vi "Test Sampling.vi"(8 "error in (no error)":errorcluster, 11 "Instrument.Lockin in":refnum<class "Instrument.Lockin.lvclass">) -> (0 "error out":errorcluster, 3 "Instrument.Lockin out":refnum<class "Instrument.Lockin.lvclass">)   [LabVIEW 2016]
uses:
  src/Instrument.Lockin/Instrument.Lockin.lvclass
  src/LockinDAQ/Typedefs/Sampling.ctl
  <vilib>/addons/_JKI Toolkits/Caraya/classes/Assert/Assert Equal Value_Variant.vi
  <userlib>/_OpenG.lib/numeric/numeric.llb/Random Number Within Range - DBL__ogtk.vi
  <vilib>/addons/_JKI Toolkits/Caraya/classes/Assert/Assert Equal Value and Type_Variant.vi
  <vilib>/addons/_JKI Toolkits/Caraya/classes/Test/Test.lvclass
  src/LockinDAQ/LockinDAQ.lvclass
  <vilib>/addons/_JKI Toolkits/Caraya/classes/Assert/Assert.lvclass
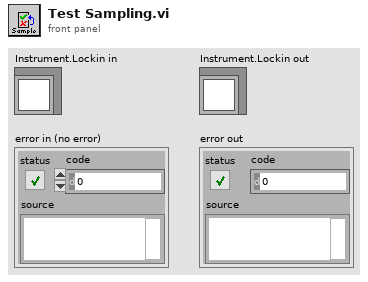
[diagram p1: front panel]
types:
  T1 = typedef "LockinDAQ.lvclass/Sampling.ctl" = cluster{"Fs":dbl, "#s":i32}
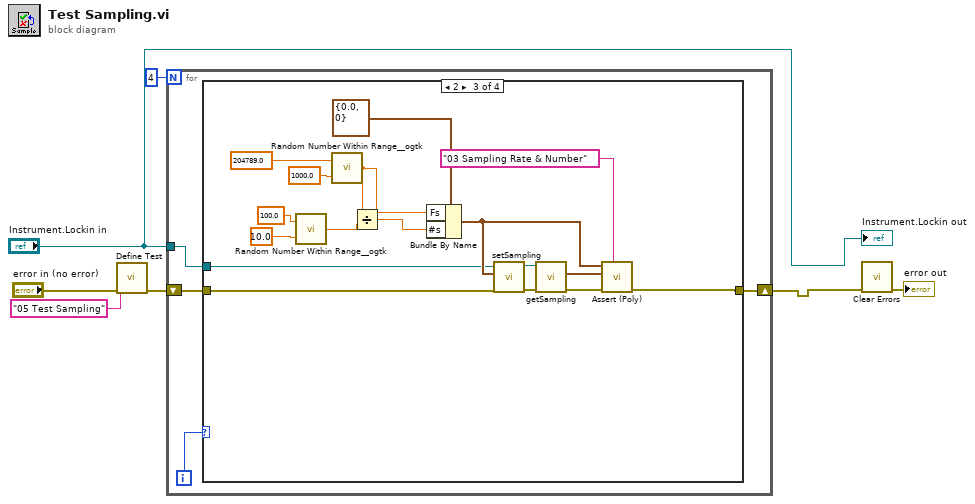
[diagram p0: block diagram]
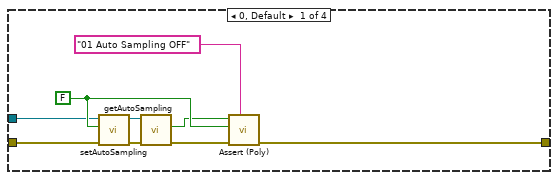
[diagram p2: hidden frame]
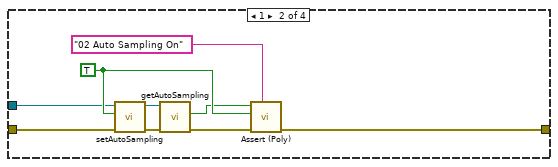
[diagram p3: hidden frame]
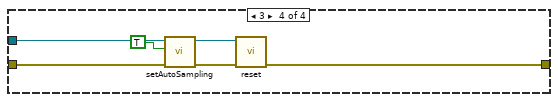
[diagram p4: hidden frame]
diagram:
  n1 = call <vilib>:"Define Test.vi"("error in (no error)"="error in (no error)", "Label (VI Title)"="05 Test Sampling") -> ("error out"=w5:errorcluster)  [unwired: 9 in]
  n2 = for {
    N: 4 -> [_]
    tunnel: "Instrument.Lockin in" -> [w9]
    shift-right: [w8] -> w4
    shift-left: w5 -> [w10]
    i -> [w11]
    n3 = case shown="2" w11 {
      tunnel: w10 -> [w13 w23 w34 w49]
      tunnel: w9 -> [w14 w22 w35 w48]
      tunnel: [w12 w21 w33 w47] -> w8
      frame 0, Default {
        w18 = FALSE ("Auto Sampling")
        n4 = call "setAutoSampling.vi"("error in (no error)"=w13, "Auto Sampling"=w18, "Instrument.Lockin in"=w14) -> ("error out"=w15:errorcluster, "Instrument.Lockin out"=w16:refnum<class "Instrument.Lockin.lvclass">)  [unwired: 7 in]
        n5 = call "getAutoSampling.vi"("error in (no error)"=w15, "Instrument.Lockin in"=w16) -> ("error out"=w19:errorcluster, "Auto Sampling"=w17:bool)  [unwired: 7 in, 1 out]
        n6 = call-poly <vilib>:"Assert (Poly).vi"("Label"="01 Auto Sampling OFF", "error in (no error)"=w19, "Y"=w18, "X"=w17) -> ("error out"=w12:errorcluster)  [unwired: 7 in]
      }
      frame 1 {
        w29 = TRUE ("Auto Sampling")
        n7 = call "setAutoSampling.vi"("error in (no error)"=w23, "Auto Sampling"=w29, "Instrument.Lockin in"=w22) -> ("error out"=w28:errorcluster, "Instrument.Lockin out"=w27:refnum<class "Instrument.Lockin.lvclass">)  [unwired: 7 in]
        n8 = call "getAutoSampling.vi"("error in (no error)"=w28, "Instrument.Lockin in"=w27) -> ("error out"=w25:errorcluster, "Auto Sampling"=w26:bool)  [unwired: 7 in, 1 out]
        n9 = call-poly <vilib>:"Assert (Poly).vi"("Label"="02 Auto Sampling On", "error in (no error)"=w25, "Y"=w29, "X"=w26) -> ("error out"=w21:errorcluster)  [unwired: 7 in]
      }
      frame 2 {
        n10 = call-poly <userlib>:"Random Number Within Range__ogtk.vi"("High"=100.0, "Low"=10.0) -> ("Random Number"=w31:dbl)  [unwired: 3 in]
        n11 = call-poly <userlib>:"Random Number Within Range__ogtk.vi"("High"=204789.0, "Low"=1000.0) -> ("Random Number"=w32:dbl)  [unwired: 3 in]
        n12 = Divide(x=w32, y=w31) -> (x/y=w30:dbl)
        n13 = Bundle By Name(cluster=T1 {"Fs"=0.0, "#s"=0} ("Sampling"), "Fs"=w32, "#s"=w30) -> (w44:T1)
        n14 = call "setSampling.vi"("error in (no error)"=w34, "Sampling"=w44, "Instrument.Lockin in"=w35) -> ("error out"=w39:errorcluster, "Instrument.Lockin out"=w40:refnum<class "Instrument.Lockin.lvclass">)  [unwired: 7 in]
        n15 = call "getSampling.vi"("error in (no error)"=w39, "Instrument.Lockin in"=w40) -> ("error out"=w37:errorcluster, "sampling"=w36:T1)  [unwired: 7 in, 1 out]
        n16 = call-poly <vilib>:"Assert (Poly).vi"("Label"="03 Sampling Rate & Number", "error in (no error)"=w37, "Y"=w36, "X"=w44) -> ("error out"=w33:errorcluster)  [unwired: 7 in]
      }
      frame 3 {
        n17 = call "setAutoSampling.vi"("error in (no error)"=w49, "Auto Sampling"=TRUE, "Instrument.Lockin in"=w48) -> ("error out"=w51:errorcluster, "Instrument.Lockin out"=w52:refnum<class "Instrument.Lockin.lvclass">)  [unwired: 7 in]
        n18 = call "reset.vi"("error in (no error)"=w51, "Instrument.Lockin in"=w52) -> ("error out"=w47:errorcluster)  [unwired: 8 in, 1 out]
      }
    }
  }
  n19 = call <vilib>:"Clear Errors.vi"("error in (no error)"=w4) -> ("error out"=→"error out":errorcluster)  [unwired: 5 in, 1 out]
  "Instrument.Lockin out" <- "Instrument.Lockin in"
